vi "Handle Autozero.vi"(8 "error in":errorcluster, 11 "Servo Switch in":refnum<class "Servo Switch.lvclass">) -> (0 "error out":errorcluster, 3 "Servo Switch out":refnum<class "Servo Switch.lvclass">)   [LabVIEW 2015, in "Open Path CRD.lvclass"]
doc: "This handles what happens when the autozero is set. When true, the switch state will be checked every iteration. While the sheath is open (SWITCH_STATE== TRUE), the fan states will be continuously monitored. When the timer trips and the sheath closes for a zero, the fans will all be turned off and the motor high time will be set to the closed value. When the timer trips again, the state of the system transitions from closed to open, the motor high time is set to the open value and the fans are reset to their original state."
uses:
  Open Path CRD.lvclass
  Switch/Servo Switch.lvclass
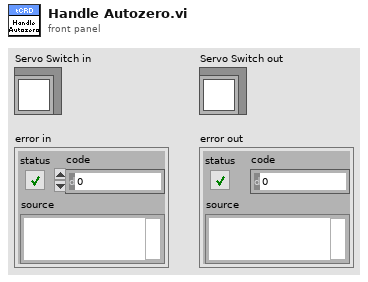
[diagram p1: front panel]
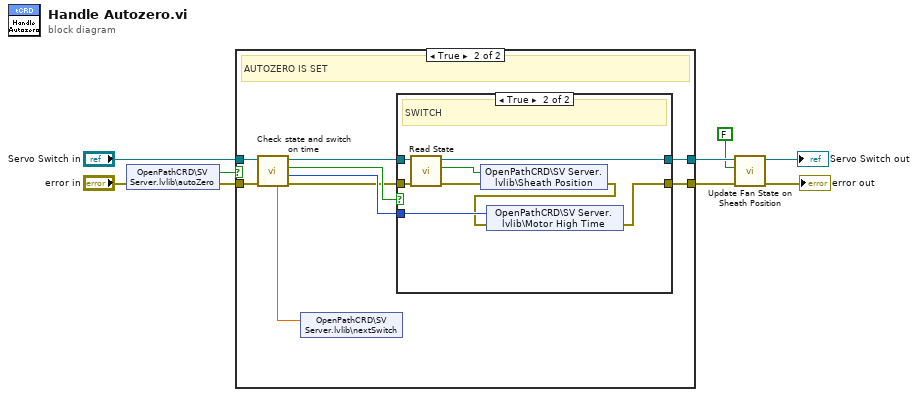
[diagram p0: block diagram]
diagram:
  n1 = shared-variable "OpenPathCRD\\SV Server.lvlib\\autoZero"(error in="error in") -> (w6:bool, error out=w9:errorcluster)
  n2 = case shown="True" w6 {
    tunnel: "Servo Switch in" -> [w11 w20]
    tunnel: [w11 w13] -> w5
    tunnel: w9 -> [w10 w17]
    tunnel: [w10 w15] -> w4
    frame False {
      # "AUTOZERO IS OFF"
    }
    frame True {
      # "AUTOZERO IS SET"
      n3 = call "Check state and switch on time.vi"("error in"=w17, "Servo Switch in"=w20) -> ("error out"=w16:errorcluster, "New Time"=w18:u32, "TimeElapsed?"=w19:bool, "Servo Switch out"=w14:refnum<class "Servo Switch.lvclass">, "NextSwitch"=w12:dbl)  [unwired: 4 in, 1 out]
      n4 = shared-variable "OpenPathCRD\\SV Server.lvlib\\nextSwitch"(w12) -> ()  [unwired: 1 in, 1 out]
      n5 = case shown="True" w19 {
        tunnel: w18 -> [_ w30]
        tunnel: w16 -> [w21 w26]
        tunnel: [w21 w29] -> w15
        tunnel: w14 -> [w22 w28]
        tunnel: [w22 w27] -> w13
        frame False {
          # "NO SWITCH"
        }
        frame True {
          # "SWITCH"
          n6 = call-dynamic "Read State.vi"("error in (no error)"=w26, "Switch in"=w28) -> ("error out"=w25:errorcluster, "State"=w23:bool, "Switch out"=w27:refnum<class "Servo Switch.lvclass">)  [unwired: 7 in]
          n7 = shared-variable "OpenPathCRD\\SV Server.lvlib\\Sheath Position"(w23, error in=w25) -> (error out=w24:errorcluster)
          n8 = shared-variable "OpenPathCRD\\SV Server.lvlib\\Motor High Time"(w30, error in=w24) -> (error out=w29:errorcluster)
        }
      }
    }
  }
  n9 = call "Update Fan State on Sheath Position.vi"("error in"=w4, "Init?"=FALSE, "Servo Switch in"=w5) -> ("error out"=→"error out":errorcluster, "Servo Switch out"=→"Servo Switch out":refnum<class "Servo Switch.lvclass">)  [unwired: 7 in]
